vi "Channels.vi"() -> (2 "Names":string[](array[string]), 3 "Channels to Create":T1[](array[typedef]) {"Custom Config Data" format="%x"})   [LabVIEW 2021, in "Template_Common.lvlib"]
uses:
  Template_Common.lvlib
  <vilib>/CIF Foundation/CIF Core/Channels/ChannelRegistrar/typedef/Channel Definition.ctl
  <vilib>/CIF Foundation/CIF Channels Core/ChannelCommon/typedef/Direction.ctl
  <vilib>/CIF Foundation/CIF Core/Channels/ChannelRegistrar/typedef/Registered Channel Types.ctl
  <vilib>/CIF Foundation/CIF Core/Channels/ChannelRegistrar/ChannelRegistrar.lvlib
  <vilib>/CIF Foundation/CIF Channels Core/ChannelCommon/ChannelCommon.lvlib
  <vilib>/CIF Foundation/CIF LabVIEW Scripting/Update Enum/Update Enum.lvlib
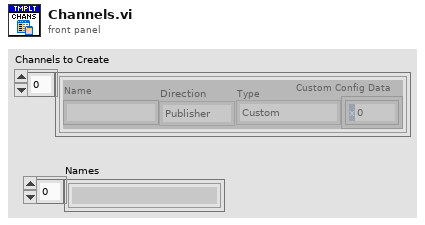
[diagram p1: front panel]
types:
  T1 = typedef "ChannelRegistrar.lvlib/Channel Definition.ctl" = cluster{"Name":string, "Direction":T2, "Type":T3, "Custom Config Data":u8[]}
  T2 = typedef "ChannelCommon.lvlib/Direction.ctl" = enum8{"Publisher", "Subscriber"}
  T3 = typedef "ChannelRegistrar.lvlib/Registered Channel Types.ctl" = enum8{"Custom", "Double_Tag", "I64_Tag", "U64_Tag", "U8_FIFO", "CAN_FIFO", "L2Enet_FIFO", "DAQ_FIFO", "Universal_FIFO", "String_Tag"}
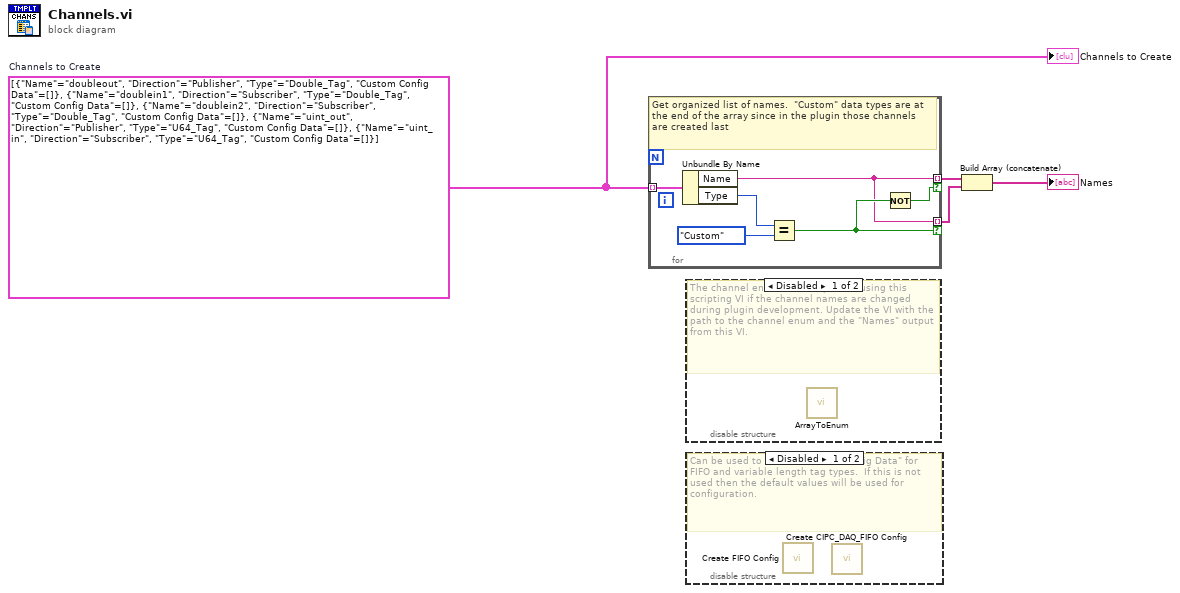
[diagram p0: block diagram]
diagram:
  w2 = T1[] [{"Name"="doubleout", "Direction"=enum."Publisher", "Type"=enum."Double_Tag", "Custom Config Data"=[]}, {"Name"="doublein1", "Direction"=enum."Subscriber", "Type"=enum."Double_Tag", "Custom Config Data"=[]}, {"Name"="doublein2", "Direction"=enum."Subscriber", "Type"=enum."Double_Tag", "Custom Config Data"=[]}, {"Name"="uint_out", "Direction"=enum."Publisher", "Type"=enum."U64_Tag", "Custom Config Data"=[]}, {"Name"="uint_in", "Direction"=enum."Subscriber", "Type"=enum."U64_Tag", "Custom Config Data"=[]}]  # Channels to Create
  n1 = for {
    tunnel: w2 -> [w10] mode=indexing
    tunnel: [w5] -> w4 mode=indexing if=w6
    tunnel: [w5] -> w3 mode=indexing if=w7
    # "Get organized list of names.  \"Custom\" data types are at the end of the array since in the plugin those channels are created last"
    n2 = Unbundle By Name(w10) -> ("Name"=w5:string, "Type"=w9:T3)
    n3 = Equal?(x=w9, y=Registered_Channel_Types."Custom") -> (x = y?=w7:bool)
    n4 = Not(x=w7) -> (.not. x?=w6:bool)
  }
  n5 = disable-structure shown="Disabled" {
    frame Disabled {
      # "The channel enum can be updated using this scripting VI if the channel names are changed during plugin development. Update the VI with the path to the channel enum and the \"Names\" output from this VI."
      n6 = call <vilib>:"ArrayToEnum.vi"() -> ()  [unwired: 11 in, 1 out]
    }
    frame Enabled {
    }
  }
  n7 = disable-structure shown="Disabled" {
    frame Disabled {
      # "Can be used to create \"Custom Config Data\" for FIFO and variable length tag types.  If this is not used then the default values will be used for configuration."
      n8 = call <vilib>:"Create FIFO Config.vi"() -> ()  [unwired: 11 in, 1 out]
      n9 = call <vilib>:"Create CIPC_DAQ_FIFO Config.vi"() -> ()  [unwired: 11 in, 1 out]
    }
    frame Enabled {
    }
  }
  n10 = Build Array (concatenate)(w4, w3) -> (→"Names":string[])
  "Channels to Create" <- w2
